vi "transmit.vi"(8 "error in (no error)":errorcluster, 11 "Subnet in":refnum<class "ISubnet.lvclass">) -> (0 "error out":errorcluster, 3 "Subnet out":refnum<class "ISubnet.lvclass">)   [LabVIEW 2015]
uses:
  Common_RT_Modbus/IModbus/IModbus.lvclass
  ISubnet.lvclass
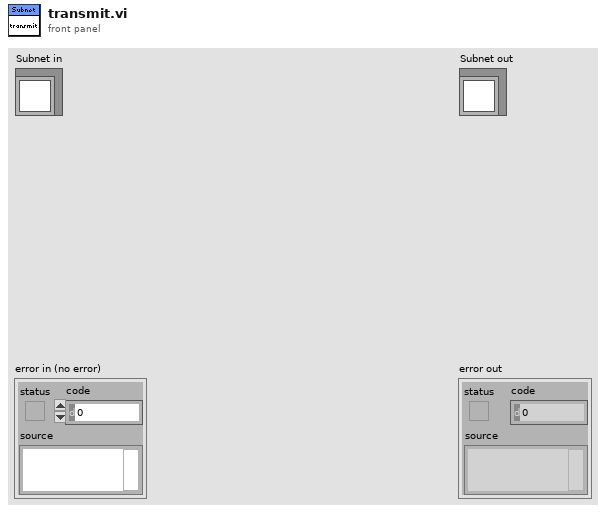
[diagram p1: front panel]
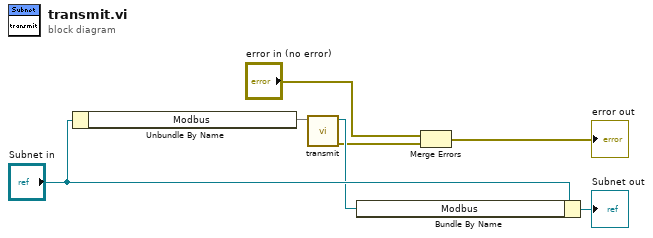
[diagram p0: block diagram]
diagram:
  n1 = Unbundle By Name("Subnet in") -> ("Modbus"=w5)
  n2 = call-dynamic "transmit.vi"("IModbus in"=w5) -> ("error out"=w3:errorcluster, "IModbus out"=w4:refnum<class "IModbus.lvclass">)  [unwired: 9 in]
  n3 = Bundle By Name(cluster="Subnet in", "Modbus"=w4) -> (→"Subnet out":refnum<class "ISubnet.lvclass">)
  n4 = Merge Errors("error in (no error)", w3) -> (→"error out":errorcluster)
